vi "UDP Vision - Sender.vi"() -> ()   [LabVIEW 2025]
doc: "The UDP protocol differs from TCP in that there is no error-checking with the packets of information that are sent, and thus no guarantee whatsoever that an intended recipient will actually receive a given piece of data.\n\nUDP does offer the ability to \"broadcast\" data across a network--simply specify an IP Address of all ones (255.255.255.255) to attempt to broadcast information network-wide. Keep in mind that routers and other network hardware will generally refuse to forward the broadcast beyond certain points, so the extent of the broadcast will in practice be limited."
uses:
  UDP Main States.ctl
  <vilib>/vision/Image Controls.llb/IMAQ Image.ctl
  94475c40-5021-47a3-af2a-3bf0d7bc5424.vi
  <vilib>/Rock Robotics/Network Tables/NT Read Integer.vi
panel:
  out "Image":T1(plugin-control)
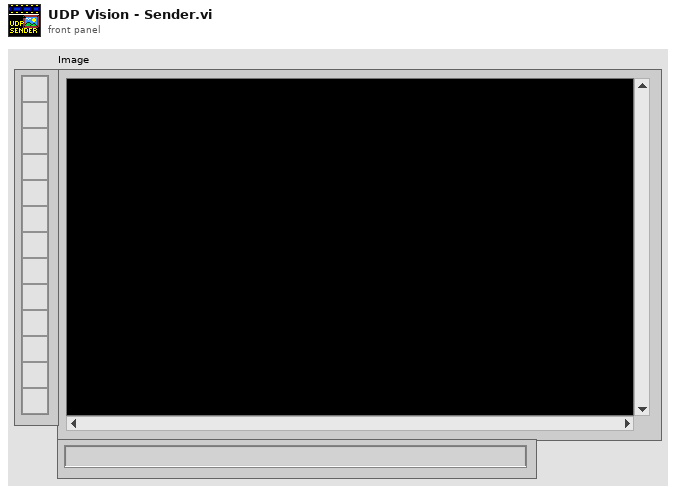
[diagram p1: front panel]
types:
  T1 = typedef "IMAQ Image.ctl" = refnum<image>
  T2 = typedef "UDP Main States.ctl" = enum16{"Message Dispatcher", "INI", "Read Data", "Send Data", "UDP Close", "UDP Open", "Exit"}
  T3 = typedef "Event Setup Types.ctl" = enum16{"Default", "Camera Loop Started", "GreyScale", "Reset Camera Settings", "Reset Team Number", "Save Data", "Setting Changed", "Update Video Mode", "Video Mode Changed", "Exit"}
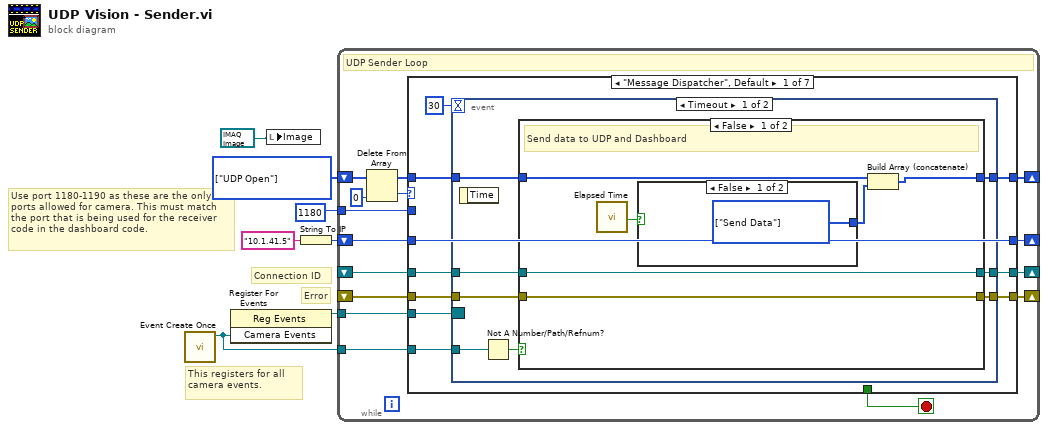
[diagram p0: block diagram]
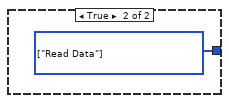
[diagram p2: hidden frame]
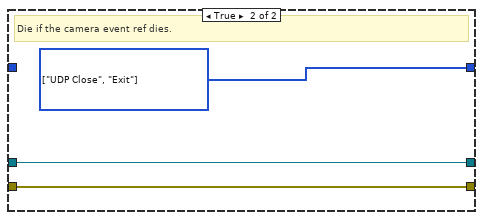
[diagram p3: hidden frame]
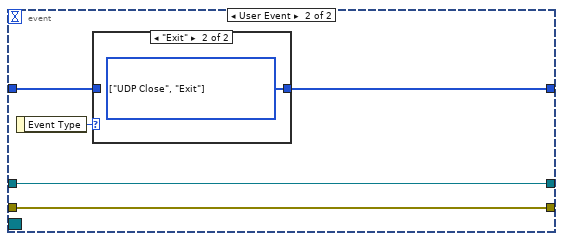
[diagram p4: hidden frame]
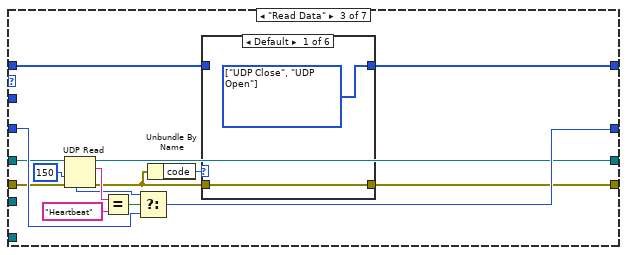
[diagram p7: hidden frame]
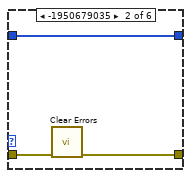
[diagram p8: hidden frame]
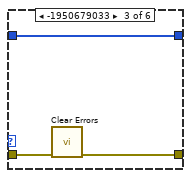
[diagram p9: hidden frame]
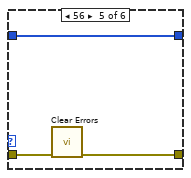
[diagram p11: hidden frame]
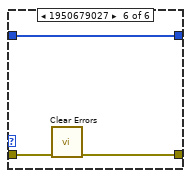
[diagram p12: hidden frame]
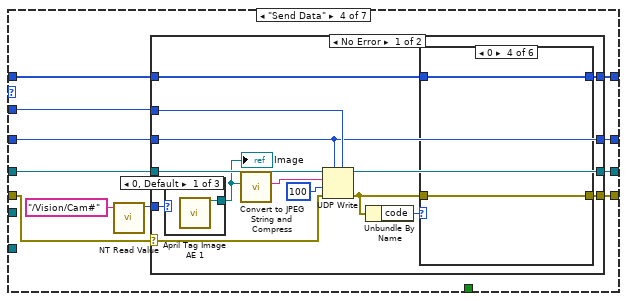
[diagram p13: hidden frame]
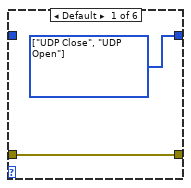
[diagram p14: hidden frame]
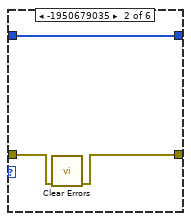
[diagram p15: hidden frame]
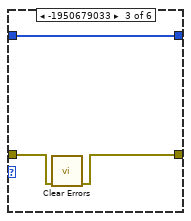
[diagram p16: hidden frame]
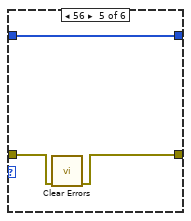
[diagram p17: hidden frame]
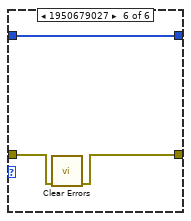
[diagram p18: hidden frame]
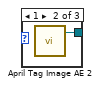
[diagram p19: hidden frame]
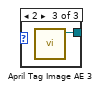
[diagram p20: hidden frame]
diagram:
  w7 = T2[] [enum."UDP Open"] items=["Message Dispatcher", "INI", "Read Data", "Send Data", "UDP Close", "UDP Open", "Exit"]
  # "Use port 1180-1190 as these are the only ports allowed for camera. This must match the port that is being used for the receiver code in the dashboard code."
  # "This registers for all camera events."
  # "Error"
  # "Connection ID"
  n1 = call "Event Create Once.vi"() -> ("Camera Events"=w3:refnum<user-event>)  [unwired: 10 in, 1 out]
  n2 = register-events(w3) -> (reference out=w5:refnum<event-registration>)  [unwired: 2 in, 1 out]
  n3 = local write "Image"(T1 refnum ("Upper Image out")) -> ()
  n4 = String To IP(1:"10.1.41.5" ("name")) -> (0:w1:u32)
  n5 = while {
    shift-right: [w17] -> _
    shift-left: w7 -> [w18]
    shift-right: [w22] -> _
    shift-left: _ -> [w20]
    shift-right: [w21] -> _
    shift-left: _ -> [w19]
    tunnel: w5 -> [w16]
    tunnel: 1180 -> [w15]
    tunnel: w3 -> [w14]
    shift-right: [w9] -> _
    shift-left: w1 -> [w8]
    stop <- w10 stop-if-true
    # "UDP Sender Loop"
    n6 = Delete From Array(array=w18, index=0) -> (deleted portion=w11:T2, array with subset deleted=w12:T2[])  [unwired: 1 in]
    n7 = case shown="\"Message Dispatcher\", Default" w11 {
      tunnel: [w32 w61 w69 w99 refnum<k16> refnum ("connection ID out") w148 w167] -> w22
      tunnel: [w31 w60 w64 w100 w141 w147 w166] -> w21
      tunnel: w20 -> [w30 w61 w68 w98 w144 _ w167]
      tunnel: w19 -> [w29 w60 w64 w101 _ _ w166]
      tunnel: [w28 w62 w65 w97 w143 w149 w165] -> w17
      tunnel: w16 -> [w27 _ _ _ _ _ _]
      tunnel: w15 -> [_ _ _ w94 _ w150 _]
      tunnel: w14 -> [w25 _ _ _ _ _ _]
      tunnel: w12 -> [w24 w62 w66 w102 w143 w151 _]
      tunnel: [_ _ _ _ _ _ TRUE] -> w10
      tunnel: [w23 w59 w71 w92 w140 w146 w164] -> w9
      tunnel: w8 -> [w23 w59 w70 w93 w140 w146 w164]
      frame "Message Dispatcher", Default {
        n8 = event shown="[0] Timeout" {
          selector: w27 -> [_ _]
          dyn-events: _ -> [_ _]
          timeout: 30 -> [_ _]
          tunnel: [w40 w55] -> w32
          tunnel: [w39 w54] -> w31
          tunnel: w30 -> [w38 w55]
          tunnel: w29 -> [w37 w54]
          tunnel: [w36 w53] -> w28
          tunnel: w25 -> [w35 _]
          tunnel: w24 -> [w33 w52]
          event Timeout {
            n9 = event-data() -> ()  [unwired: 1 in, 1 out]
            n10 = Not A Number/Path/Refnum?(number/path/refnum=w35) -> (NaN/Path/Refnum?=w34:bool)
            n11 = case shown="False" w34 {
              tunnel: [w43 w50] -> w40
              tunnel: [w44 w49] -> w39
              tunnel: w38 -> [w43 w50]
              tunnel: w37 -> [w44 w49]
              tunnel: w33 -> [w46 _]
              tunnel: [w45 w51] -> w36
              frame False {
                # "Send data to UDP and Dashboard"
                n12 = call "Elapsed Time"() -> ("Time has Elapsed"=w41:bool)  [unwired: 12 in, 7 out]
                n13 = case shown="False" w41 {
                  tunnel: [w47 w48] -> w42
                  frame False {
                    w47 = T2[] [enum."Send Data"] items=["Message Dispatcher", "INI", "Read Data", "Send Data", "UDP Close", "UDP Open", "Exit"]
                  }
                  frame True {
                    w48 = T2[] [enum."Read Data"] items=["Message Dispatcher", "INI", "Read Data", "Send Data", "UDP Close", "UDP Open", "Exit"]
                  }
                }
                n14 = Build Array (concatenate)(w46, w42) -> (w45:T2[])
              }
              frame True {
                w51 = T2[] [enum."UDP Close", enum."Exit"] items=["Message Dispatcher", "INI", "Read Data", "Send Data", "UDP Close", "UDP Open", "Exit"] ("value out")
                # "Die if the camera event ref dies."
              }
            }
          }
          event User Event {
            n15 = event-data() -> ("Event Type"=w56:T3)  [unwired: 1 in]
            n16 = case shown="\"Exit\"" w56 {
              tunnel: w52 -> [w57 _]
              tunnel: [w57 w58] -> w53
              frame Default {
              }
              frame "Exit" {
                w58 = T2[] [enum."UDP Close", enum."Exit"] items=["Message Dispatcher", "INI", "Read Data", "Send Data", "UDP Close", "UDP Open", "Exit"]
              }
            }
          }
        }
      }
      frame "INI" {
      }
      frame "Read Data" {
        n17 = UDP Read(connection ID=w68, timeout ms (25000)=150) -> (data out=w75:string, 3:w69:refnum<k16>, 6:w72:u32)  [unwired: 2 in, 2 out]
        n18 = Equal?(x=w75, y="Heartbeat" ("data in")) -> (x = y?=w73:bool)
        n19 = Select(t=w72, s=w73, f=w70) -> (s? t:f=w71:i64)
        n20 = Unbundle By Name(w64) -> ("code"=w63:i32)
        n21 = case shown="Default" w63 {
          tunnel: [w77 w79 w82 w85 w87 w90] -> _
          tunnel: w64 -> [w77 w80 w83 w85 w88 w91]
          tunnel: w66 -> [_ w78 w81 w84 w86 w89]
          tunnel: [w76 w78 w81 w84 w86 w89] -> w65
          frame Default {
            w76 = T2[] [enum."UDP Close", enum."UDP Open"] items=["Message Dispatcher", "INI", "Read Data", "Send Data", "UDP Close", "UDP Open", "Exit"]
          }
          frame -1950679035 {
            n22 = call <vilib>:"Clear Errors.vi"("error in (no error)"=w80) -> ("error out"=w79:errorcluster)  [unwired: 5 in, 1 out]
          }
          frame -1950679033 {
            n23 = call <vilib>:"Clear Errors.vi"("error in (no error)"=w83) -> ("error out"=w82:errorcluster)  [unwired: 5 in, 1 out]
          }
          frame 0 {
          }
          frame 56 {
            n24 = call <vilib>:"Clear Errors.vi"("error in (no error)"=w88) -> ("error out"=w87:errorcluster)  [unwired: 5 in, 1 out]
          }
          frame 1950679027 {
            n25 = call <vilib>:"Clear Errors.vi"("error in (no error)"=w91) -> ("error out"=w90:errorcluster)  [unwired: 5 in, 1 out]
          }
        }
      }
      frame "Send Data" {
        n26 = call-poly <vilib>:"NT Read Value.vi"("name"="/Vision/Cam#" ("Name")) -> ("value"=w95:i64)  [unwired: 8 in, 2 out]
        n27 = case shown="No Error" w101 {
          selector: w101 -> [w114 w138]
          tunnel: [w108 w138] -> w100
          tunnel: [w116 w139] -> w99
          tunnel: w98 -> [w115 w139]
          tunnel: w95 -> [w113 w136]
          tunnel: w102 -> [w105 _]
          tunnel: [w104 w137] -> w97
          tunnel: w94 -> [w110 _]
          tunnel: w93 -> [w103 _]
          tunnel: [w103 w136] -> w92
          frame No Error {
            n28 = case shown="0, Default" w113 {
              tunnel: [w133 w134 w135] -> w112
              frame 0, Default {
                n29 = call "April Tag Image AE 1.vi"() -> ("Apriltag Image out"=w133:T1)  [unwired: 11 in]
              }
              frame 1 {
                n30 = call "April Tag Image AE 2.vi"() -> ("Apriltag Image out"=w134:T1)  [unwired: 11 in]
              }
              frame 2 {
                n31 = call "April Tag Image AE 3.vi"() -> ("Apriltag Image out"=w135:T1)  [unwired: 11 in]
              }
            }
            "Image" <- w112
            n32 = call "Convert to JPEG String and Compress.vi"("Image"=w112) -> ("JPEG Image String"=w111:string)  [unwired: 10 in]
            n33 = UDP Write(address=w103, port or service name=w110, connection ID=w115, data in=w111, 8:w114, 9:100 ("timeout ms (25000)")) -> (error out=w106:errorcluster, 3:w116:refnum<k16>)
            n34 = Unbundle By Name(w106) -> ("code"=w107:i32)
            n35 = case shown="0" w107 {
              tunnel: [w118 w120 w123 w126 w128 w131] -> w108
              tunnel: w106 -> [w118 w121 w124 w126 w129 w132]
              tunnel: w105 -> [_ w119 w122 w125 w127 w130]
              tunnel: [w117 w119 w122 w125 w127 w130] -> w104
              frame Default {
                w117 = T2[] [enum."UDP Close", enum."UDP Open"] items=["Message Dispatcher", "INI", "Read Data", "Send Data", "UDP Close", "UDP Open", "Exit"]
              }
              frame -1950679035 {
                n36 = call <vilib>:"Clear Errors.vi"("error in (no error)"=w121) -> ("error out"=w120:errorcluster)  [unwired: 5 in, 1 out]
              }
              frame -1950679033 {
                n37 = call <vilib>:"Clear Errors.vi"("error in (no error)"=w124) -> ("error out"=w123:errorcluster)  [unwired: 5 in, 1 out]
              }
              frame 0 {
              }
              frame 56 {
                n38 = call <vilib>:"Clear Errors.vi"("error in (no error)"=w129) -> ("error out"=w128:errorcluster)  [unwired: 5 in, 1 out]
              }
              frame 1950679027 {
                n39 = call <vilib>:"Clear Errors.vi"("error in (no error)"=w132) -> ("error out"=w131:errorcluster)  [unwired: 5 in, 1 out]
              }
            }
          }
          frame Error {
            w137 = T2[] [enum."UDP Close", enum."UDP Open"] items=["Message Dispatcher", "INI", "Read Data", "Send Data", "UDP Close", "UDP Open", "Exit"]
          }
        }
      }
      frame "UDP Close" {
        n40 = UDP Close(connection ID=w144) -> (error out=w145:errorcluster)  [unwired: 1 in, 1 out]
        n41 = call <vilib>:"Clear Errors.vi"("error in (no error)"=w145) -> ("error out"=w141:errorcluster)  [unwired: 5 in, 1 out]
      }
      frame "UDP Open" {
        n42 = UDP Open(8:errorcluster {"status"=FALSE, "code"=0, "source"=""} ("error in (no error)"), 9:1000 ("timeout ms (wait forever: -1)"), 11:w150) -> (port=w155:refnum<k16>, 0:w152:errorcluster)  [unwired: 2 in, 1 out]
        n43 = case shown="No Error" w152 {
          selector: w152 -> [w158 w162]
          tunnel: [w158 w162] -> w147
          tunnel: w151 -> [w157 _]
          tunnel: [w157 w160] -> w149
          tunnel: w155 -> [w156 w161]
          tunnel: [w156 w161] -> w148
          frame No Error {
          }
          frame Error {
            w163 = T2[] [enum."UDP Close", enum."UDP Open"] items=["Message Dispatcher", "INI", "Read Data", "Send Data", "UDP Close", "UDP Open", "Exit"]
            # "If there is an error opening, try closing than reopening after 2 seconds."
            n44 = call "Stall Data Flow.vim"("value in"=w163, "milliseconds to wait"=u32 2000) -> ("value out"=w160:T2[])  [unwired: 1 out]
          }
        }
      }
      frame "Exit" {
        w165 = T2[] [] items=["Message Dispatcher", "INI", "Read Data", "Send Data", "UDP Close", "UDP Open", "Exit"] ("value out")
      }
    }
  }
